vi "CleanUp.vi"(0 "ActionLvDialog in":refnum<class "ActionLvDialog.lvclass">, 5 "error in (no error)":errorcluster) -> (14 "ActionLvDialog out":refnum<class "ActionLvDialog.lvclass">, 19 "error out":errorcluster)   [LabVIEW 2017, in "ActionLvDialog.lvclass"]
doc: "Base class implementation (empty)."
uses:
  ActionLvDialog.lvclass
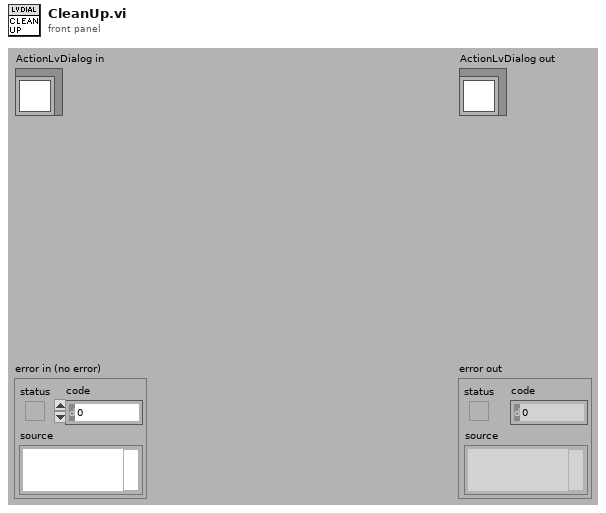
[diagram p1: front panel]
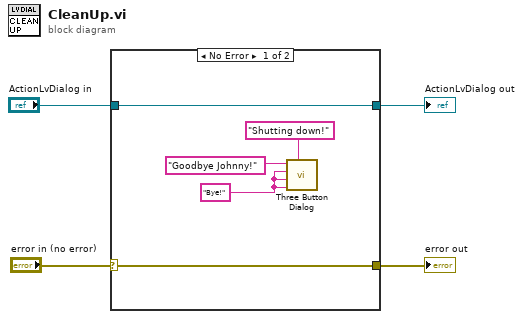
[diagram p0: block diagram]
diagram:
  n1 = case shown="No Error" "error in (no error)" {
    selector: "error in (no error)" -> [w6 w10]
    tunnel: "ActionLvDialog in" -> [w5 w11]
    tunnel: [w6 w10] -> w2
    tunnel: [w5 w11] -> w1
    frame No Error {
      w7 = "Bye!" ("Left Button Text (\"Yes\")")
      n2 = call <vilib>:"Three Button Dialog.vi"("Window Title (\"\")"="Shutting down!" ("Window Title (\"\")"), "Right Button Text (\"Cancel\")"=w7, "Center Button Text (\"No\")"=w7, "Left Button Text (\"Yes\")"=w7, "message"="Goodbye Johnny!") -> ()  [unwired: 6 in, 1 out]
    }
    frame Error {
    }
  }
  "error out" <- w2
  "ActionLvDialog out" <- w1
